vi "Coding_morse4.vi"() -> ()   [LabVIEW 2022 SP3]
uses:
  <vilib>/sound2/lvsound2.llb/Sampling Mode.ctl
  <vilib>/sound2/lvsound2.llb/Sound Data Format.ctl
panel:
  in  "Alphabet":string[][](array[string])=[["a", ".-"], ["b", "-..."], ["c", "-.-."], ["d", "-.."], ["e", "."], ["f", "..-."], ["g", "--."], ["h", "...."], ["i", ".."], ["j", ".---"], ["k", "-.-"], ["l", ".-.."], ["m", "--"], ["n", "-."], ["o", "---"], ["p", ".--."], ["q", "--.-"], ["r", ".-."], ["s", "..."], ["t", "-"], ["u", "..-"], ["v", "...-"], ["w", ".--"], ["x", "-..-"], ["y", "-.--"], ["z", "--.."], ["1", ".----"], ["2", "..---"], ["3", "...--"], ["4", "....-"], ["5", "....."], ["6", "-...."], ["7", "--..."], ["8", "---.."], ["9", "----."], ["0", "-----"], [" ", "space"]]
  in  "Input Words words":string="o propozitie cu ceva"
  out "Whole code":string[](array[string])
  in  "Dit time(ms)":dbl=200.0
  in  "Volume":dbl(knob) scale=0.0..100.0
  in  "Frequency":dbl=4000.0
  out "Character code remained":i32
  out "current dit/dash time":dbl
  out "String":string
  out "Current code":string
  out "Waiting until next word":bool
  in  "stop":bool
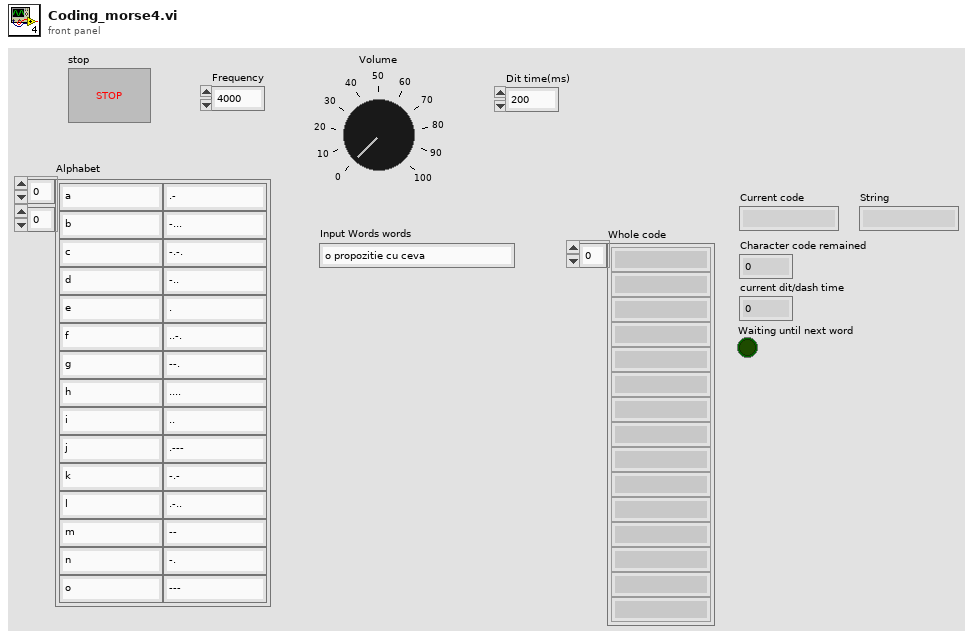
[diagram p1: front panel]
types:
  T1 = typedef "Sound Data Format.ctl" = cluster{"sample rate (S/s)":dbl, "number of channels":i32, "bits per sample":i32}
  T2 = typedef "Sampling Mode.ctl" = i32
  T3 = typedef "Sound Output Task ID.ctl" = u32
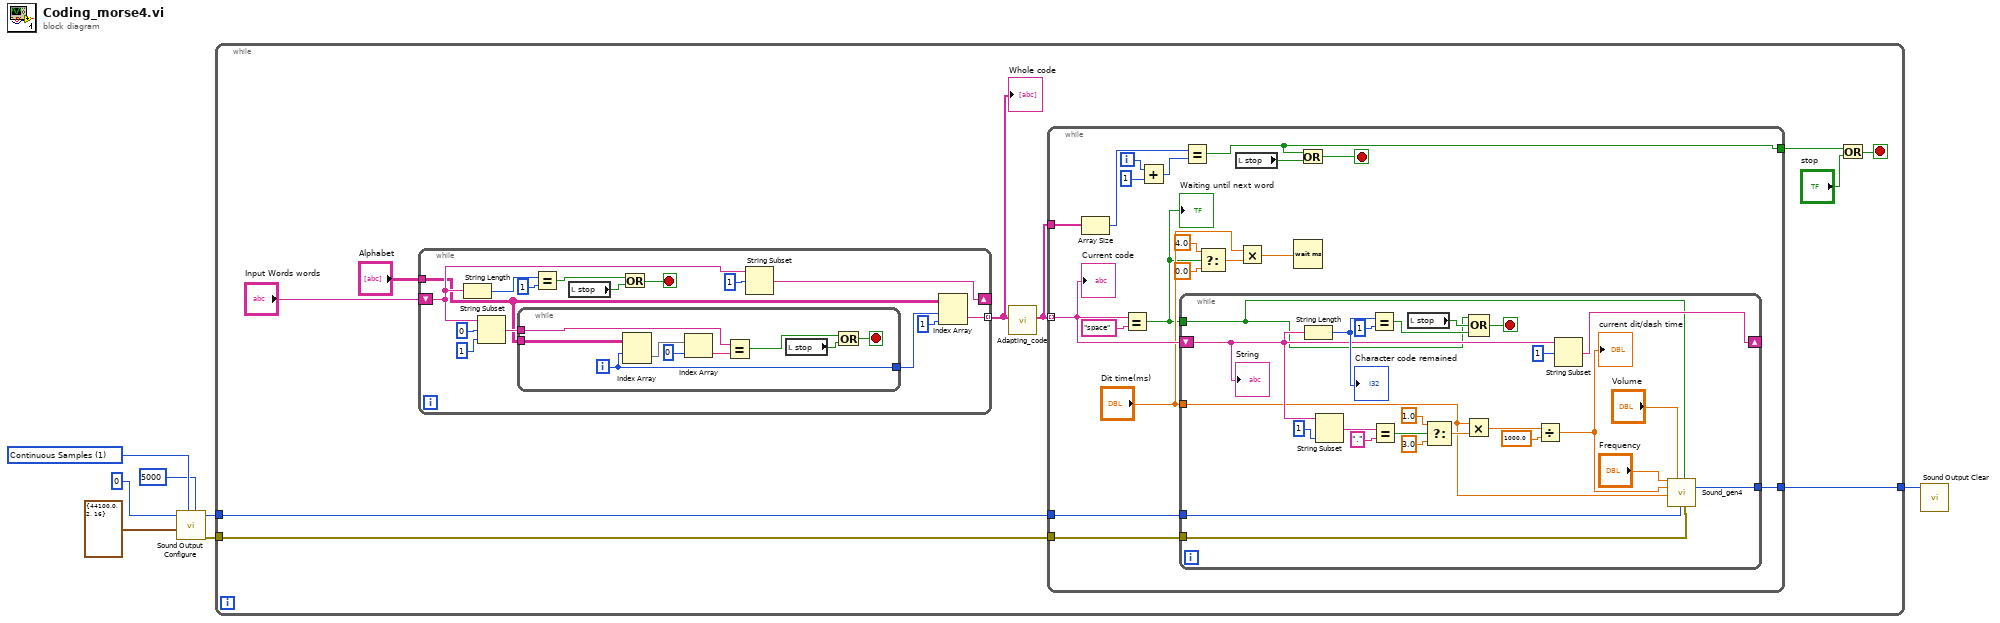
[diagram p0: block diagram]
diagram:
  w5 = T2 1 items=["Finite Samples", "Continuous Samples"] ("sample mode")
  n1 = call <vilib>:"Sound Output Configure.vi"("number of samples/ch"=5000, "sample mode"=w5, "sound format"=T1 {"sample rate (S/s)"=44100.0, "number of channels"=2, "bits per sample"=16}, "device ID"=u32 0) -> ("error out"=w3:errorcluster, "task ID"=w2:T3)  [unwired: 6 in]
  n2 = while {
    tunnel: w3 -> [w12]
    tunnel: w2 -> [w11]
    tunnel: [w10] -> w1
    stop <- w13 stop-if-true
    n3 = while {
      shift-right: [w70] -> _
      shift-left: "Input Words words" -> [w71]
      tunnel: "Alphabet" -> [w67]
      tunnel: [w62] -> w8 mode=indexing
      stop <- w63 stop-if-true
      n4 = String Length(string=w71) -> (length=w64:i32)
      n5 = String Subset(string=w71, offset (0)=0, length (rest)=1 ("length (rest)")) -> (substring=w68:string)
      n6 = while {
        tunnel: w67 -> [w85]
        tunnel: w68 -> [w82]
        tunnel: [w77] -> w66
        i -> [w77]
        stop <- w78 stop-if-true
        n7 = Index Array(array=w85, index (row)=w77) -> (element=w83:string[])  [unwired: 1 in]
        n8 = Index Array(array=w83, index=0) -> (element=w81:string)
        n9 = Equal?(x=w82, y=w81) -> (x = y?=w80:bool)
        n10 = local read "stop"() -> (w79:bool)
        n11 = Or(x=w80, y=w79) -> (x .or. y?=w78:bool)
      }
      n12 = Equal?(x=w64, y=1) -> (x = y?=w74:bool)
      n13 = local read "stop"() -> (w75:bool)
      n14 = Or(x=w74, y=w75) -> (x .or. y?=w63:bool)
      n15 = String Subset(string=w71, offset (0)=1) -> (substring=w70:string)  [unwired: 1 in]
      n16 = Index Array(array=w67, index (row)=w66, index (col)=1 ("disabled index (col)")) -> (element=w62:string)
    }
    "Whole code" <- w8
    n17 = call "Adapting_code.vi"("Code"=w8) -> ("Code with an extra dot"=w9:string[])  [unwired: 10 in]
    n18 = while {
      tunnel: w9 -> [w28] mode=indexing
      tunnel: w9 -> [w33]
      tunnel: [w35] -> w15
      tunnel: w12 -> [w20]
      tunnel: w11 -> [w19]
      tunnel: [w18] -> w10
      i -> [w31]
      stop <- w34 stop-if-true
      n19 = Array Size(array=w33) -> (size(s)=w32:i32)
      n20 = Equal?(x=w28, y="space") -> (x = y?=w21:bool)
      "Waiting until next word" <- w21
      n21 = Add(x=w31, y=1) -> (x+y=w29:i32)
      n22 = while {
        shift-right: [w48] -> _
        shift-left: w28 -> [w50]
        tunnel: "Dit time(ms)" -> [w47]
        tunnel: w21 -> [w37]
        tunnel: w20 -> [w43]
        tunnel: w19 -> [w42]
        tunnel: [w41] -> w18
        stop <- w38 stop-if-true
        n23 = String Length(string=w50) -> (length=w61:i32)
        "Character code remained" <- w61
        n24 = String Subset(string=w50, length (rest)=1 ("length (rest)")) -> (substring=w59:string)  [unwired: 1 in]
        n25 = Equal?(x=w61, y=1) -> (x = y?=w39:bool)
        n26 = Equal?(x=w59, y=".") -> (x = y?=w58:bool)
        n27 = local read "stop"() -> (w40:bool)
        n28 = Select(t=1.0, s=w58, f=3.0) -> (s? t:f=w60:dbl)
        n29 = Multiply(x=w47, y=w60) -> (x*y=w53:dbl)
        n30 = Compound Arithmetic op=OR(w37, w40, w39) -> (w38:bool)
        n31 = Divide(x=w53, y=1000.0) -> (x/y=w45:dbl)
        "current dit/dash time" <- w45
        n32 = String Subset(string=w50, offset (0)=1) -> (substring=w48:string)  [unwired: 1 in]
        n33 = call "Sound_gen4.vi"("Frequency"="Frequency", "Sound time(s)"=w45, "Dit time(ms)"=w47, "Volume"="Volume", "task ID"=w42, "Is space"=w37, "error in (no error)"=w43) -> ("task ID out"=w41:T3)  [unwired: 19 in, 1 out]
        "String" <- w50
      }
      n34 = Equal?(x=w32, y=w29) -> (x = y?=w35:bool)
      n35 = Select(t=4.0, s=w21, f=0.0) -> (s? t:f=w24:dbl)
      n36 = local read "stop"() -> (w36:bool)
      n37 = Multiply(x="Dit time(ms)", y=w24) -> (x*y=w22:dbl)
      n38 = Wait (ms)(milliseconds to wait=w22) -> ()  [unwired: 1 out]
      n39 = Or(x=w35, y=w36) -> (x .or. y?=w34:bool)
      "Current code" <- w28
    }
    n40 = Or(x=w15, y="stop") -> (x .or. y?=w13:bool)
  }
  n41 = call <vilib>:"Sound Output Clear.vi"("task ID"=w1) -> ()  [unwired: 10 in, 1 out]
